vi "Agilent N934X Series Configure and Query Marker.vi"() -> ()   [LabVIEW 2022 SP3]
doc: "This example shows how to configure the spectrum analyzer to query marker."
uses:
  <instrlib>/Agilent N934X Series/Public/Configure/Configure Frequency (Start Stop).vi
  <instrlib>/Agilent N934X Series/Agilent N934X Series.lvlib
panel:
  in  "Marker Mode (0: Position)":i32(ring) items=["Position", "Delta", "Off"]
  in  "Detector Type(0: Negative Peak)":i32(ring) items=["Negative Peak", "Positive Peak", "Sample", "Average", "Normal"]
  in  "Stop Frequency (7E+9 Hz)":dbl=7000000000.0
  in  "Start Frequency (9E+3 Hz)":dbl=9000.0
  in  "Measurement Type (0: Spectrum Analyzer)":i32(ring) items=["Spectrum Analyzer", "Tracking Generator", "Power Meter", "Modulation Analyzer", "Reflection Measurement"]
  in  "VISA resource name":refnum<visa-resource-name>
  out "Marker Position":dbl
  in  "Active Marker (1: Marker1)":i32(ring)=1 items=["Marker1"=1, "Marker2"=2, "Marker3"=3, "Marker4"=4, "Marker5"=5, "Marker6"=6, "Marker7"=7, "Marker8"=8, "Marker9"=9, "Marker10"=10, "Marker11"=11, "Marker12"=12]
  in  "Marker Search (0: Maximum)":u16(ring) items=["Maximum", "Next Peak", "Next Peak Left", "Next Peak Right", "Minimum", "Peak to Peak"]
  in  "Reference Level (0 dBm)":dbl
  in  "Reference Level Offset (0 dB)":dbl
  # "(c) 2012-2025 National Instruments.  ALL RIGHTS RESERVED."
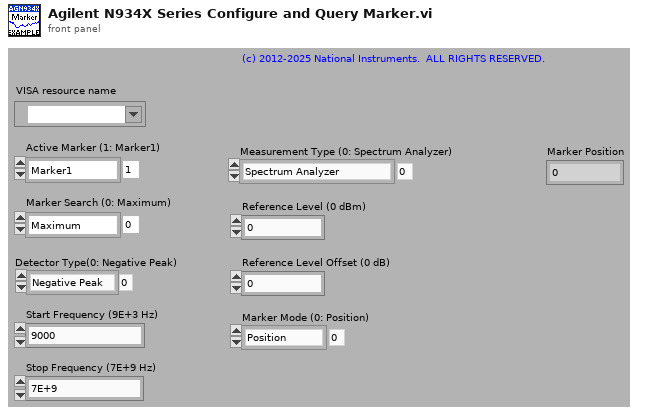
[diagram p1: front panel]
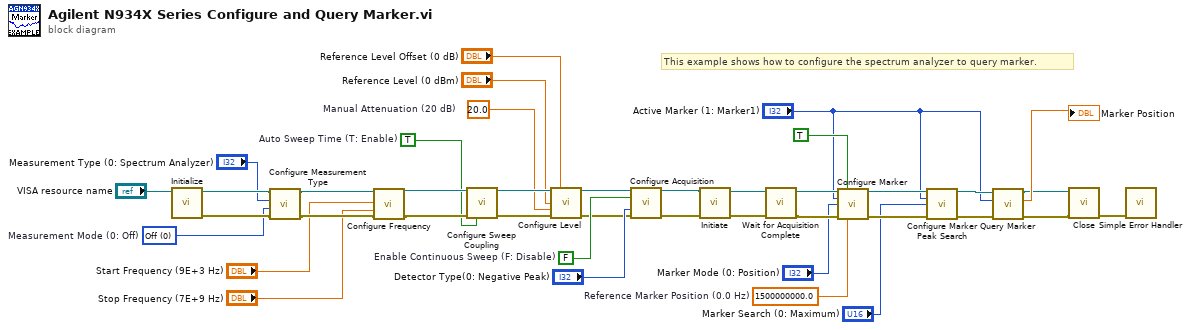
[diagram p0: block diagram]
diagram:
  w1 = 20.0  # Manual Attenuation (20 dB)
  w2 = 0 items=["Off", "Channel Power Measurement", "Adjacent Channel Power Ratio Measurement", "Occupied Bandwidth Measurement", "Spectrum Monitor", "Spectrum Emission Mask", "Channel Scanner", "AM Measurement", "ASK Measurement", "FM Measurement", "FSK Measurement"]  # Measurement Mode (0: Off)
  w14 = 1500000000.0  # Reference Marker Position (0.0 Hz)
  w30 = TRUE  # Auto Sweep Time (T: Enable)
  w25 = FALSE  # Enable Continuous Sweep (F: Disable)
  # "This example shows how to configure the spectrum analyzer to query marker."
  n1 = call <instrlib>:"Initialize.vi"("VISA resource name"="VISA resource name") -> ("error out"=w39:errorcluster, "VISA resource name out"=w38:refnum<visa-resource-name>)  [unwired: 9 in]
  n2 = call <instrlib>:"Configure Measurement Type.vi"("error in (no error)"=w39, "Measurement Mode (0: Off)"=w2, "Measurement Type (0: Spectrum Analyzer)"="Measurement Type (0: Spectrum Analyzer)", "VISA resource name"=w38) -> ("error out"=w35:errorcluster, "VISA resource name out"=w36:refnum<visa-resource-name>)  [unwired: 6 in]
  n3 = call-poly <instrlib>:"Configure Frequency.vi"("VISA resource name"=w36, "Start Frequency (9E+3 Hz)"="Start Frequency (9E+3 Hz)", "error in (no error)"=w35, "Stop Frequency (7E+9 Hz)"="Stop Frequency (7E+9 Hz)") -> ("VISA resource name out"=w32:refnum<visa-resource-name>, "error out"=w31:errorcluster)  [unwired: 10 in]
  n4 = call <instrlib>:"Configure Sweep Coupling.vi"("VISA resource name"=w32, "error in (no error)"=w31, "Auto Video Bandwidth (T: Enable)"=w30) -> ("VISA resource name out"=w29:refnum<visa-resource-name>, "error out"=w28:errorcluster)  [unwired: 11 in]
  n5 = call <instrlib>:"Configure Level.vi"("VISA resource name"=w29, "Reference Level Offset (0 dB)"="Reference Level Offset (0 dB)", "Reference Level (0 dBm)"="Reference Level (0 dBm)", "Manual Attenuation (20 dB)"=w1, "error in (no error)"=w28) -> ("VISA resource name out"=w23:refnum<visa-resource-name>, "error out"=w22:errorcluster)  [unwired: 9 in]
  n6 = call <instrlib>:"Configure Acquisition.vi"("VISA resource name"=w23, "Enable Continuous Sweep(F: Disable)"=w25, "Detector Type(0: Negative Peak)"="Detector Type(0: Negative Peak)", "error in (no error)"=w22) -> ("VISA resource name out"=w21:refnum<visa-resource-name>, "error out"=w20:errorcluster)  [unwired: 10 in]
  n7 = call <instrlib>:"Initiate.vi"("error in (no error)"=w20, "VISA resource name"=w21) -> ("error out"=w19:errorcluster, "VISA resource name out"=w18:refnum<visa-resource-name>)  [unwired: 8 in]
  n8 = call <instrlib>:"Wait for Acquisition Complete.vi"("error in (no error)"=w19, "VISA resource name"=w18) -> ("error out"=w17:errorcluster, "VISA resource name out"=w16:refnum<visa-resource-name>)  [unwired: 8 in]
  n9 = call <instrlib>:"Configure Marker.vi"("VISA resource name"=w16, "Enable Marker (T: Enable)"=TRUE, "Active Marker (1: Marker 1)"="Active Marker (1: Marker1)", "Marker Mode (0: Position)"="Marker Mode (0: Position)", "error in (no error)"=w17, "Marker Position (5E+6 Hz)"=w14) -> ("VISA resource name out"=w11:refnum<visa-resource-name>, "error out"=w12:errorcluster)  [unwired: 8 in]
  n10 = call <instrlib>:"Configure Marker Peak Search.vi"("VISA resource name"=w11, "Active Marker (1: Marker 1)"="Active Marker (1: Marker1)", "Marker Search (0: Maximum)"="Marker Search (0: Maximum)", "error in (no error)"=w12) -> ("VISA resource name out"=w9:refnum<visa-resource-name>, "error out"=w8:errorcluster)  [unwired: 10 in]
  n11 = call <instrlib>:"Query Marker.vi"("error in (no error)"=w8, "Active Marker (1: Marker 1)"="Active Marker (1: Marker1)", "VISA resource name"=w9) -> ("error out"=w5:errorcluster, "Y Value"=→"Marker Position":dbl, "VISA resource name out"=w4:refnum<visa-resource-name>)  [unwired: 6 in]
  n12 = call <instrlib>:"Close.vi"("error in (no error)"=w5, "VISA resource name"=w4) -> ("error out"=w3:errorcluster)  [unwired: 9 in]
  n13 = call <vilib>:"Simple Error Handler.vi"("error in (no error)"=w3) -> ()  [unwired: 1 in, 8 out]
